vi "Table ROI exit.vi"(9 "List Parameter Fit In":dbl[][](array[numeric]), 10 "List ROI In":dbl[][](array[numeric]), 11 "Table In":string[][](table)) -> (3 "Table Out":string[][](table))   [LabVIEW 2023]
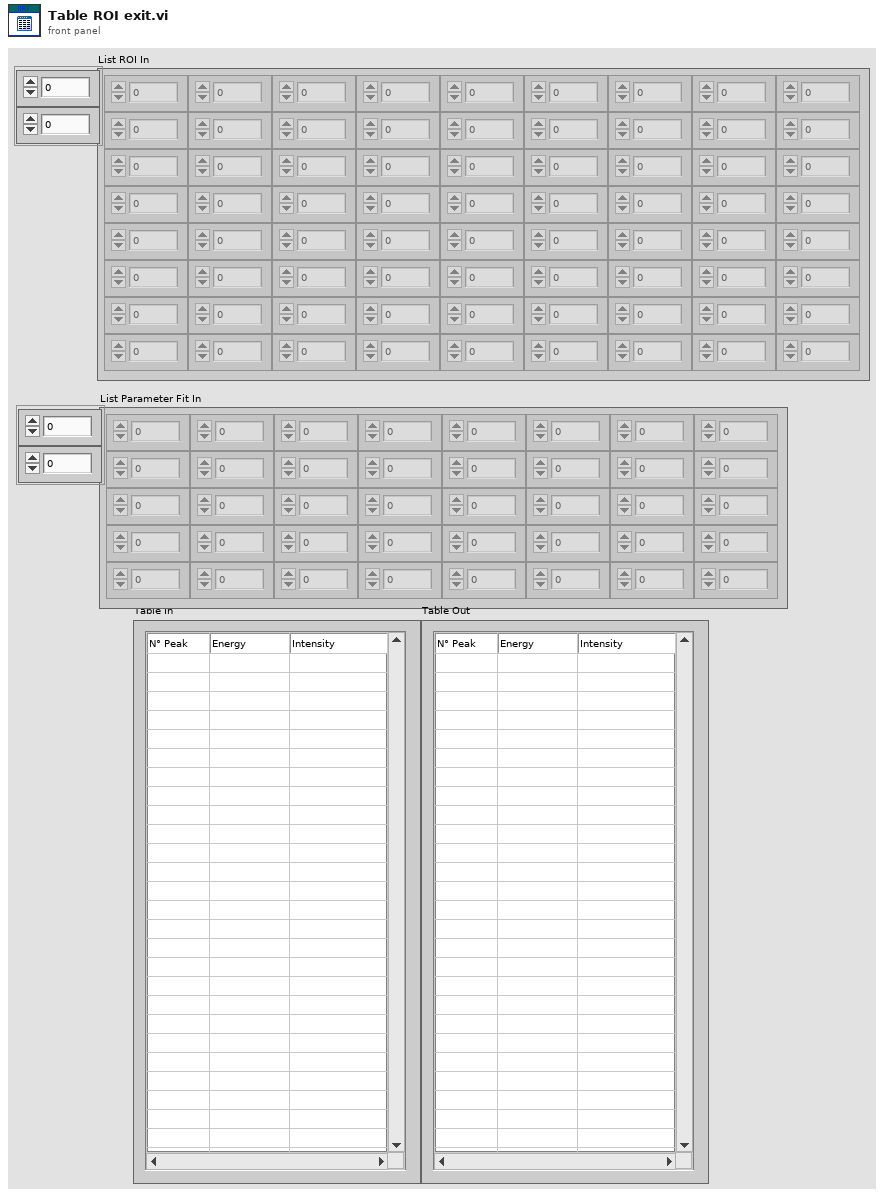
[diagram p1: front panel]
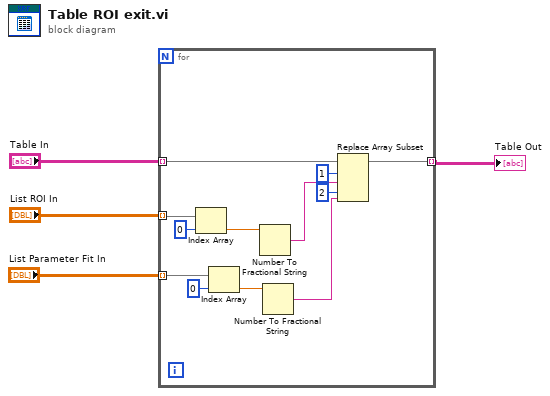
[diagram p0: block diagram]
diagram:
  n1 = for {
    tunnel: "Table In" -> [w16] mode=indexing
    tunnel: "List ROI In" -> [w15] mode=indexing
    tunnel: "List Parameter Fit In" -> [w9] mode=indexing
    tunnel: [w5] -> w1 mode=indexing
    n2 = Index Array(array=w15, index=0) -> (element=w12:dbl)
    n3 = Index Array(array=w9, index=0) -> (element=w8:dbl)
    n4 = Number To Fractional String(number=w12) -> (F-format string=w11:string)  [unwired: 3 in]
    n5 = Number To Fractional String(number=w8) -> (F-format string=w7:string)  [unwired: 3 in]
    n6 = Replace Array Subset(array=w16, new element #1=w11, index #1=1 ("index"), new element #2=w7, index #2=2 ("index")) -> (w5:string[])
  }
  "Table Out" <- w1
